vi "64x128OLED_SSD1315.vi"() -> ()   [LabVIEW 2024]
uses:
  Driver/Public/Digital Pull Direction.ctl
  a7562c57-8a3f-42dc-a248-a218528d61d2.vi
  Public/InitialiseOLED.vi
  Public/GetPicture.vi
  Public/BuildMessagesFromPicture.vi
  Driver/CTIPicoVISA.lvlib
  OLEDI2CMessageGenerator.lvlib
panel:
  out "Numeric":i32
  in  "stop":bool
  out "2D Picture":picture
  in  "Grove Connector":enum16{"I2C0", "I2C1"}(ring)
  out "Identity":T1
  out "error out":errorcluster={"status"=TRUE, "code"=15, "source"="CTI.lvlib:Session.lvclass:Check I2C Pins.vi:4130001<ERR>\nInvalid pin selection for I2C:\nGPIO 5 is invalid for I2C 1 SCL, valid options: 3, 7, 11, 15, 19, 27\r\nGPIO 4 is invalid for I2C 1 SDA, valid options: 2, 6, 10, 14, 18, 26\n\n\n<b>Complete call chain:</b>\r\n     CTI.lvlib:Session.lvclass:Check I2C Pins.vi:4130001\r\n     CTI.lvlib:Session.lvclass:Reserve I2C.vi\r\n     CTI.lvlib:Session.lvclass:Configure I2C.vi:7080001\r\n     I2CLCD1602.vi"}
  in  "Port":refnum<visa-resource-name>="COM7"
  # "https://wiki.seeedstudio.com/Grove-OLED-Display-0.96-SSD1315/"
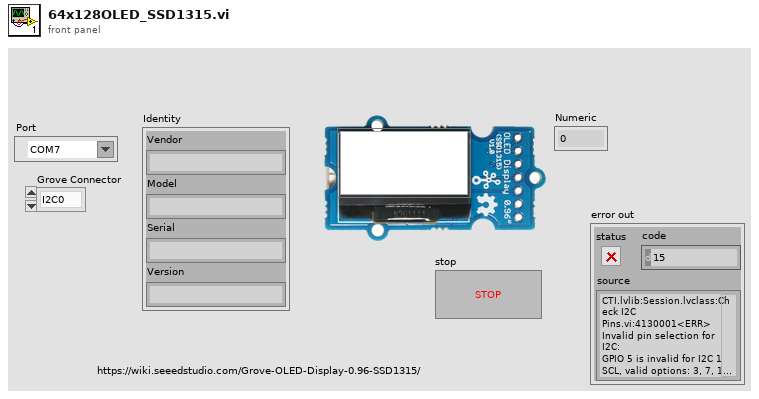
[diagram p1: front panel]
types:
  T1 = cluster{"Vendor":string, "Model":string, "Serial":string, "Version":string}
  T2 = cluster{"Font Name:":string, "Size":i16, "Strikeout?":bool, "Italic?":bool, "Underline?":bool, "Outline?":bool, "Shadow?":bool, "Bold?":bool}
  T3 = typedef "CTIPicoVISA.lvlib/Digital Pull Direction.ctl" = enum16{"None", "Up", "Down", "Both"}
  T4 = enum16{"User-specified Font", "Application Font", "System Font", "Dialog Font"}
  T5 = cluster{"horizontal":enum16{"left", "center", "right"}, "vertical":enum16{"top", "center", "bottom"}}
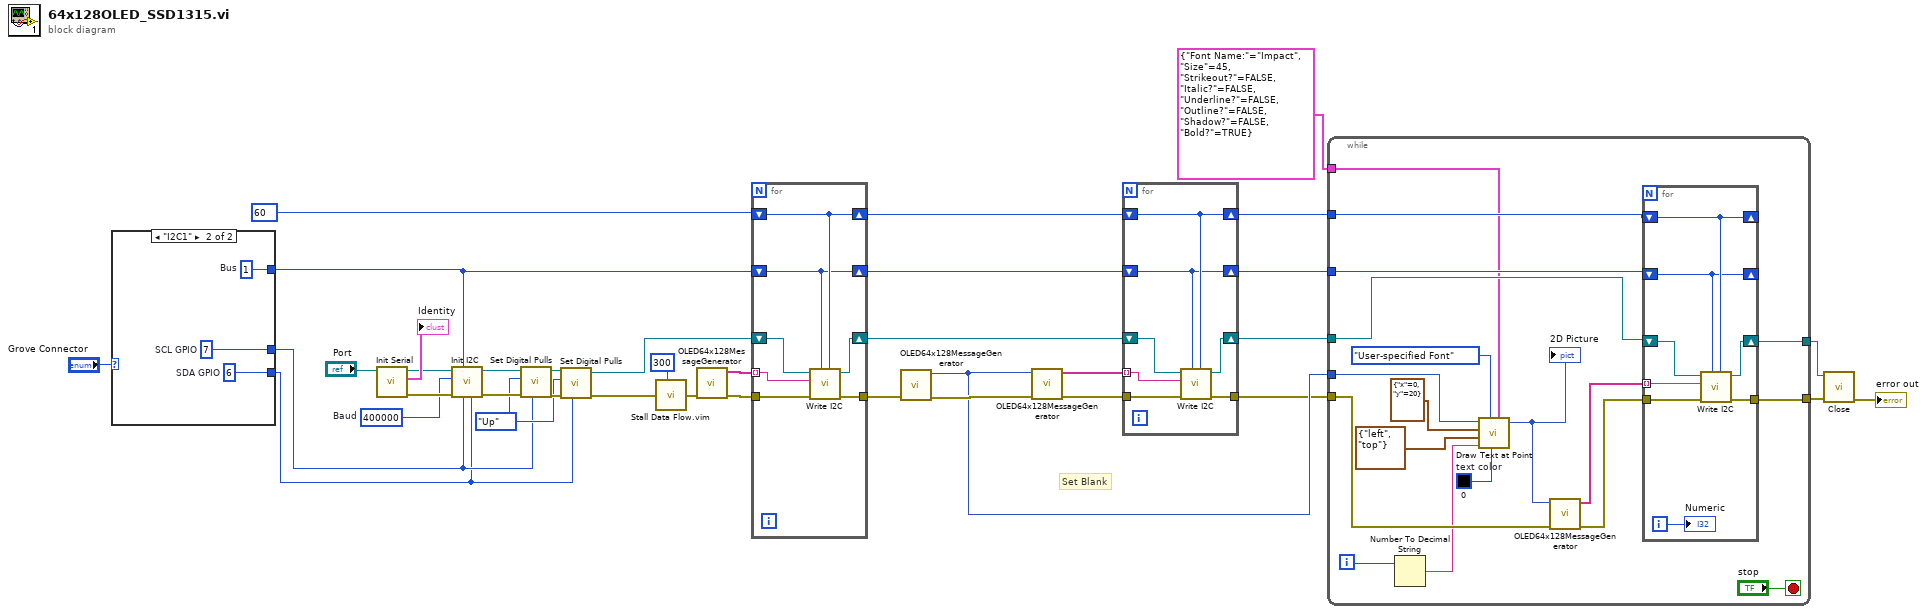
[diagram p0: block diagram]
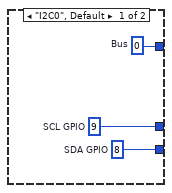
[diagram p2: hidden frame]
diagram:
  w28 = Digital_Pull_Direction."Up" ("Pull")
  w23 = u32 400000  # Baud
  # "Set Blank"
  n1 = case shown="\"I2C1\"" "Grove Connector" {
    tunnel: [w40 w43] -> w15
    tunnel: [w39 w42] -> w14
    tunnel: [w38 w41] -> w21
    frame "I2C0", Default {
      w38 = u8 0  # Bus
      w39 = 8  # SDA GPIO
      w40 = 9  # SCL GPIO
    }
    frame "I2C1" {
      w41 = u8 1  # Bus
      w42 = 6  # SDA GPIO
      w43 = 7  # SCL GPIO
    }
  }
  n2 = call "Init Serial.vi"("VISA resource name in"="Port") -> ("error out"=w24:errorcluster, "Identity"=→"Identity":T1, "VISA resource name Out"=w25:refnum<visa-resource-name>)  [unwired: 8 in]
  n3 = call "Init I2C.vi"("SDA GPIO"=w14, "SCL GPIO"=w15, "Bus"=w21, "error in (no error)"=w24, "Baud"=w23, "VISA resource name in"=w25) -> ("error out"=w31:errorcluster, "VISA resource name"=w32:refnum<visa-resource-name>)  [unwired: 4 in]
  n4 = call "Set Digital Pulls.vi"("GPIO"=w15, "error in (no error)"=w31, "Pull"=w28, "VISA resource name in"=w32) -> ("error out"=w29:errorcluster, "VISA resource name"=w30:refnum<visa-resource-name>)  [unwired: 6 in]
  n5 = call "Set Digital Pulls.vi"("GPIO"=w14, "error in (no error)"=w29, "Pull"=w28, "VISA resource name in"=w30) -> ("error out"=w11:errorcluster, "VISA resource name"=w10:refnum<visa-resource-name>)  [unwired: 6 in]
  n6 = call "Stall Data Flow.vim"("value in"=w11, "milliseconds to wait"=u32 300) -> ("value out"=w26:errorcluster)  [unwired: 1 out]
  n7 = call-poly "OLED64x128MessageGenerator.vi"("error in (no error)"=w26) -> ("error out"=w22:errorcluster, "Messages"=w33:string[])  [unwired: 9 in]
  n8 = for {
    tunnel: w33 -> [w48] mode=indexing
    tunnel: w22 -> [w50]
    tunnel: [w47] -> w19
    shift-right: [w46] -> w5
    shift-left: w10 -> [w49]
    shift-right: [w45] -> w6
    shift-left: u8 60 ("Address") -> [w45]
    shift-right: [w44] -> w4
    shift-left: w21 -> [w44]
    n9 = call "Write I2C.vi"("Address"=w45, "Bus"=w44, "error in (no error)"=w50, "Data"=w48, "VISA resource name in"=w49) -> ("error out"=w47:errorcluster, "VISA resource name"=w46:refnum<visa-resource-name>)  [unwired: 5 in]
  }
  n10 = call-poly "OLED64x128MessageGenerator.vi"("error in (no error)"=w19) -> ("error out"=w13:errorcluster, "2D Picture"=w12:picture)  [unwired: 9 in]
  n11 = call-poly "OLED64x128MessageGenerator.vi"("error in (no error)"=w13, "2D Picture"=w12) -> ("error out"=w9:errorcluster, "Messages"=w8:string[])  [unwired: 8 in]
  n12 = for {
    tunnel: w8 -> [w55] mode=indexing
    tunnel: w9 -> [w57]
    tunnel: [w54] -> w7
    shift-right: [w53] -> w3
    shift-left: w5 -> [w56]
    shift-right: [w52] -> w1
    shift-left: w6 -> [w52]
    shift-right: [w51] -> w2
    shift-left: w4 -> [w51]
    n13 = call "Write I2C.vi"("Address"=w52, "Bus"=w51, "error in (no error)"=w57, "Data"=w55, "VISA resource name in"=w56) -> ("error out"=w54:errorcluster, "VISA resource name"=w53:refnum<visa-resource-name>)  [unwired: 5 in]
  }
  n14 = while {
    tunnel: w12 -> [w75]
    tunnel: w7 -> [w71]
    tunnel: w1 -> [w70]
    tunnel: w2 -> [w69]
    tunnel: w3 -> [w68]
    tunnel: [w65] -> w17
    tunnel: [w58] -> w18
    tunnel: T2 {"Font Name:"="Impact", "Size"=45, "Strikeout?"=FALSE, "Italic?"=FALSE, "Underline?"=FALSE, "Outline?"=FALSE, "Shadow?"=FALSE, "Bold?"=TRUE} ("[user-specified font]") -> [w61]
    i -> [w62]
    stop <- "stop" stop-if-true
    w72 = u32 0  # text color
    n15 = Number To Decimal String(number=w62) -> (decimal integer string=w59:string)  [unwired: 1 in]
    n16 = call <vilib>:"Draw Text at Point.vi"("[user-specified font]"=w61, "text color(black)"=w72, "desired font(Application)"=T4."User-specified Font", "text"=w59, "alignment(left, top)"=T5 {"horizontal"=enum."left", "vertical"=enum."top"}, "origin"=cluster{"x":i16, "y":i16} {"x"=0, "y"=20}, "picture"=w75) -> ("new picture"=w63:picture)  [unwired: 3 in, 1 out]
    "2D Picture" <- w63
    n17 = call-poly "OLED64x128MessageGenerator.vi"("error in (no error)"=w71, "2D Picture"=w63) -> ("error out"=w67:errorcluster, "Messages"=w66:string[])  [unwired: 8 in]
    n18 = for {
      tunnel: w66 -> [w81] mode=indexing
      tunnel: w67 -> [w83]
      tunnel: [w80] -> w58
      shift-right: [w79] -> w65
      shift-left: w68 -> [w82]
      shift-right: [w78] -> _
      shift-left: w70 -> [w78]
      shift-right: [w77] -> _
      shift-left: w69 -> [w77]
      i -> [w76]
      n19 = call "Write I2C.vi"("Address"=w78, "Bus"=w77, "error in (no error)"=w83, "Data"=w81, "VISA resource name in"=w82) -> ("error out"=w80:errorcluster, "VISA resource name"=w79:refnum<visa-resource-name>)  [unwired: 5 in]
      "Numeric" <- w76
    }
  }
  n20 = call "Close.vi"("error in (no error)"=w18, "VISA resource name in"=w17) -> ("error out"=→"error out":errorcluster)  [unwired: 9 in]
